vi "Replace_Possibly_Stat_Dots_to_Trees-2.vi"(0 "[IN] Possibly\nMoving (X,Y)":dbl[][](array[numeric]), 1 "[IN] Stationary Dots":T1(array[cluster]), 2 "[IN] Dot matrix after using \nsome filters which contains \ndots with increased statuses":i16[][](array[numeric]), 3 "error IN":errorcluster, 4 "[IN] dR min":dbl, 5 "Closing gaps":i32 min=1) -> (7 "[OUT] Stationary Dots":T1(array[cluster]), 8 "[OUT] Dot matrix after using \nsome filters which contains \ndots with increased statuses":i16[][](array[numeric]), 9 "error OUT":errorcluster)   [LabVIEW 2013]
panel:
  out "Number of dots \nwith changing status":i32
  out "Number of\nallocations":i32
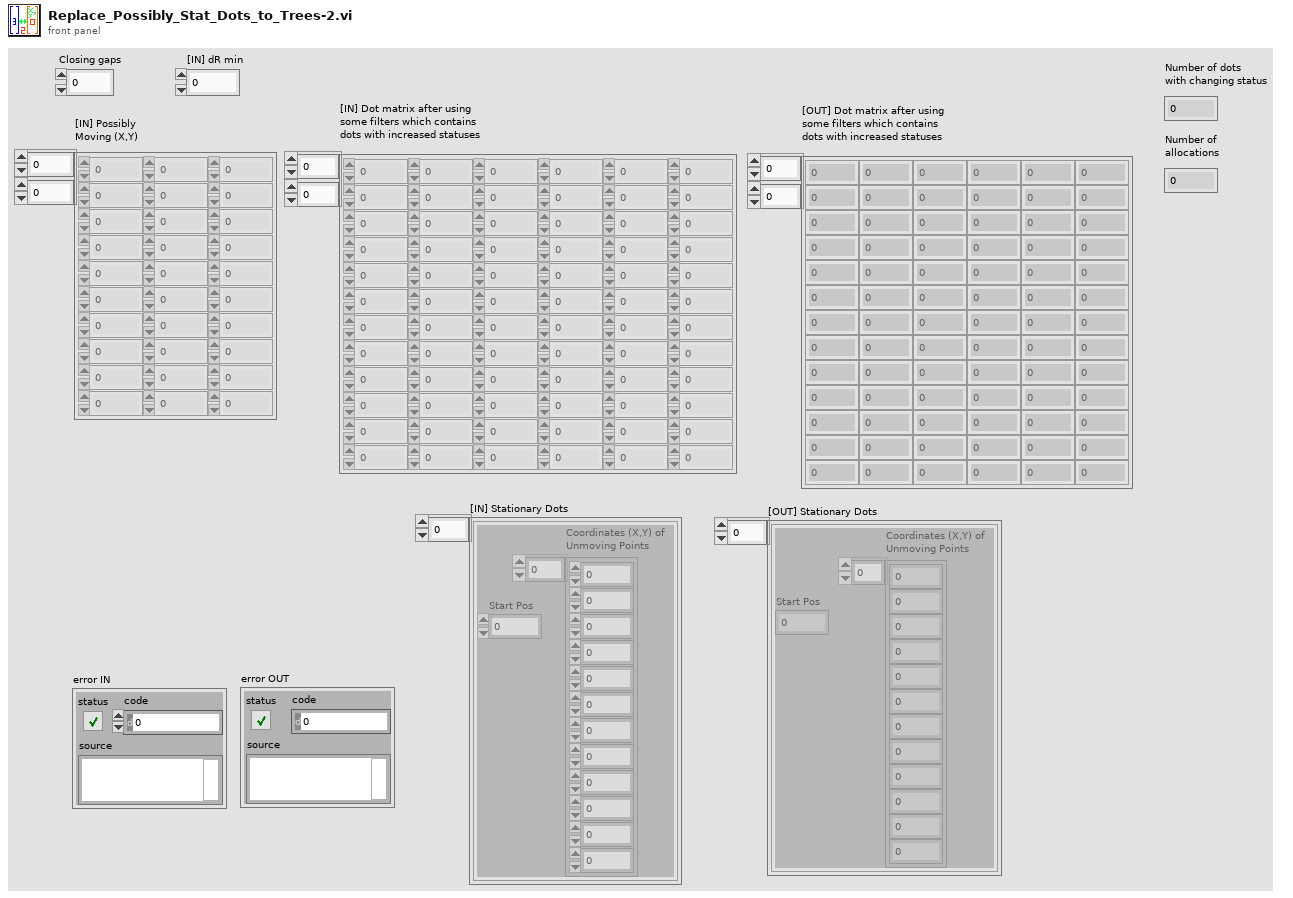
[diagram p1: front panel]
types:
  T1 = cluster{"Coordinates (X,Y) of\nUnmoving Points":dbl[], "Start Pos":i32}[]
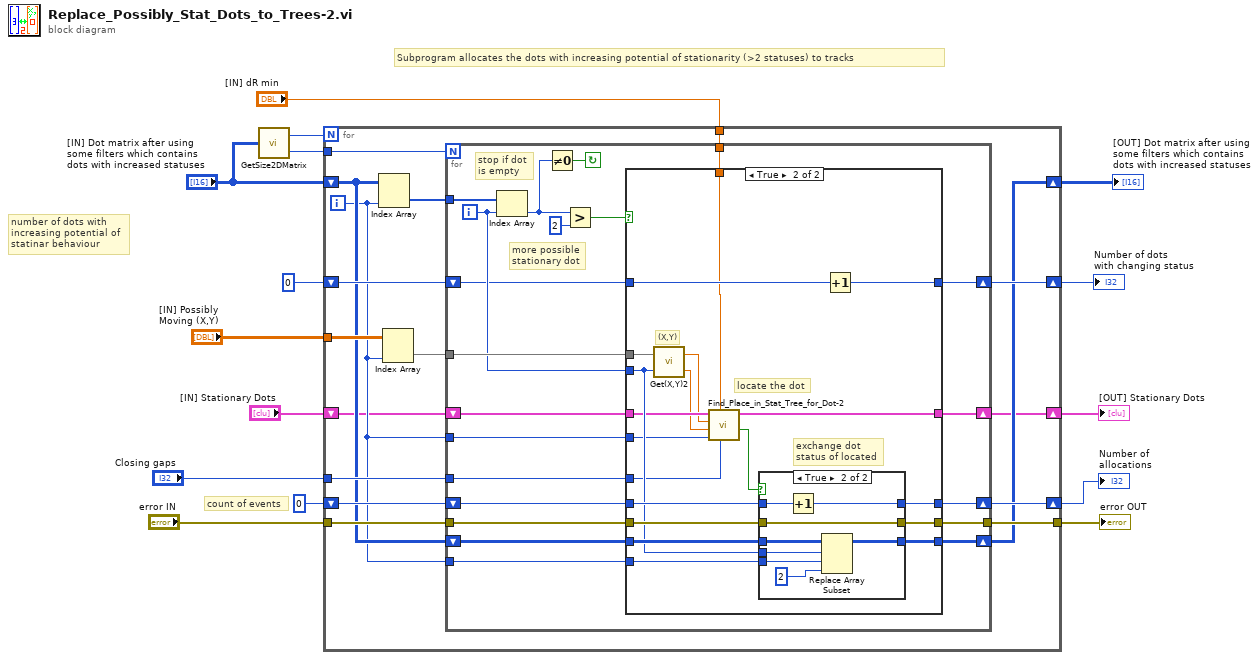
[diagram p0: block diagram]
diagram:
  # "number of dots with \nincreasing potential of\nstatinar behaviour"
  # "count of events"
  # "Subprogram allocates the dots with increasing potential of stationarity (>2 statuses) to tracks"
  n1 = call "GetSize2DMatrix.vi"("Array IN (2D)"="[IN] Dot matrix after using \nsome filters which contains \ndots with increased statuses") -> ("# Cols"=w15:i32, "# Rows"=w14:i32)
  n2 = for {
    N: w15 -> [_]
    tunnel: w14 -> [w32]
    tunnel: "[IN] Possibly\nMoving (X,Y)" -> [w30]
    tunnel: "[IN] dR min" -> [w28]
    tunnel: "Closing gaps" -> [w27]
    shift-right: [w25] -> w7
    shift-left: 0 -> [w26]
    tunnel: "error IN" -> [w24]
    tunnel: [w23] -> w8
    shift-right: [w21] -> w5
    shift-left: 0 -> [w22]
    shift-right: [w18] -> w3
    shift-left: "[IN] Dot matrix after using \nsome filters which contains \ndots with increased statuses" -> [w20]
    shift-right: [w16] -> w1
    shift-left: "[IN] Stationary Dots" -> [w17]
    i -> [w19]
    n3 = Index Array(array=w20, index (col)=w19) -> (element=w31:i16[])  [unwired: 1 in]
    n4 = Index Array(array=w30, index (col)=w19) -> (element=w29:dbl[])  [unwired: 1 in]
    n5 = for {
      N: w32 -> [_]
      tunnel: w31 -> [w53]
      tunnel: w29 -> [w48]
      tunnel: w28 -> [w46]
      tunnel: w19 -> [w45]
      tunnel: w27 -> [w44]
      shift-right: [w42] -> w25
      shift-left: w26 -> [w43]
      tunnel: w24 -> [w41]
      tunnel: [w40] -> w23
      shift-right: [w38] -> w21
      shift-left: w22 -> [w39]
      shift-right: [w35] -> w18
      shift-left: w20 -> [w37]
      tunnel: w19 -> [w36]
      shift-right: [w33] -> w16
      shift-left: w17 -> [w34]
      i -> [w47]
      stop <- w52 continue-if-true
      # "more possible\nstationary dot"
      # "stop if dot\nis empty"
      n6 = Index Array(array=w53, index=w47) -> (element=w51:i16)
      n7 = Not Equal To 0?(x=w51) -> (x != 0?=w52:bool)
      n8 = Greater?(x=w51, y=i16 2) -> (0:w49:bool)
      n9 = case shown="True" w49 {
        tunnel: w48 -> [_ w77]
        tunnel: w47 -> [_ w68]
        tunnel: w46 -> [_ w64]
        tunnel: w45 -> [_ w60]
        tunnel: w44 -> [_ w59]
        tunnel: w43 -> [w58 w76]
        tunnel: [w58 w75] -> w42
        tunnel: w41 -> [w57 w74]
        tunnel: [w57 w73] -> w40
        tunnel: w39 -> [w56 w72]
        tunnel: [w56 w71] -> w38
        tunnel: w37 -> [w55 w70]
        tunnel: w36 -> [_ w69]
        tunnel: [w55 w67] -> w35
        tunnel: w34 -> [w54 w63]
        tunnel: [w54 w65] -> w33
        frame False {
        }
        frame True {
          # "locate the dot"
          # "exchange dot \nstatus of located"
          # "(X,Y)"
          n10 = call "Get(X,Y)2.vi"("[IN] index of (X,Y)"=w68, "[IN] Array coordi\nnates (X,Y) in Frame"=w77) -> ("[OUT] Y"=w61:dbl, "[OUT] X"=w62:dbl)
          n11 = call "Find_Place_in_Stat_Tree_for_Dot-2.vi"("[IN] Closing gaps"=w59, "[IN] dR min"=w64, "# frame = \nindex of dot"=w60, "Y"=w61, "X"=w62, "[IN] Stationary Dots"=w63) -> ("Potential unmoving \ndot is allocated"=w66:bool, "[OUT] Stationary Dots \nwith Additional Points"=w65:T1)  [unwired: 2 in]
          n12 = case shown="True" w66 {
            tunnel: w76 -> [w80 w88]
            tunnel: [w80 w87] -> w75
            tunnel: w74 -> [w79 w86]
            tunnel: [w79 w86] -> w73
            tunnel: w70 -> [w78 w85]
            tunnel: w69 -> [_ w81]
            tunnel: w68 -> [_ w82]
            tunnel: [w78 w83] -> w67
            frame False {
            }
            frame True {
              n13 = Increment(x=w88) -> (x+1=w87:i32)
              n14 = Replace Array Subset(array=w85, new element=i16 2, index (row)=w82, index (col)=w81) -> (w83:i16[][])
            }
          }
          n15 = Increment(x=w72) -> (x+1=w71:i32)
        }
      }
    }
  }
  "error OUT" <- w8
  "Number of\nallocations" <- w7
  "[OUT] Dot matrix after using \nsome filters which contains \ndots with increased statuses" <- w3
  "Number of dots \nwith changing status" <- w5
  "[OUT] Stationary Dots" <- w1
